vi "NewBusNumber.vi"(8 "ErrorArray In":errorcluster[](array[cluster]), 10 "clFrontPanelControlRefs In":T1) -> (0 "ErrorArray Out":errorcluster[](array[cluster]), 1 "BusNumber":u8, 2 "clFrontPanelControlRefs Out":T1)   [LabVIEW 2014, in "TestFramework.lvlib"]
uses:
  TestFramework.lvlib
  TypeDefs/clFrontPanelControlRefs.ctl
  FGenPlugins/MyPluginBaseClass/TypeDef/PluginParams.ctl
  WfrmGenerator/WfrmPlugins/EventPluginBaseClass/TypeDefs/dblEvtSignalArray.ctl
  FGenPlugins/MyPluginBaseClass/TypeDef/CreateArbWfrmParams.ctl
  WfrmGenerator/WfrmPlugins/EventPluginBaseClass/TypeDefs/clEvtConfig.ctl
  WfrmGenerator/WfrmModule/PublicAPI/Arguments/Requests/dblEvtParams.ctl
  FGenPlugins/MyPluginBaseClass/TypeDef/ConfigArbWfrmParams.ctl
  FGenPlugins/MyPluginBaseClass/TypeDef/TriggerParams.ctl
  <vilib>/Utility/error.llb/Error Cluster From Error Code.vi
  <vilib>/ErrorRing/Error Ring.xnode
  <userlib>/NIST/NISTErrorLib/NISTErrorLib.lvlib
  FGenPlugins/MyPluginBaseClass/NISTFGenPluginsBase.lvclass
  WfrmGenerator/WfrmPlugins/EventPluginBaseClass/BaseWfrmPlugin.lvclass
  WfrmGenerator/WfrmModule/WfrmModule.lvlib
panel:
  # "When you add a control \non the front panel, add a\nreference for it in this\ntype def.  This cluster\nwill hold all of the refer-\nences to the front panel\ncontrols in order to pass\nthese control references \nto subvis."
  # "When you add a control \non the front panel, add a\nreference for it in this\ntype def.  This cluster\nwill hold all of the refer-\nences to the front panel\ncontrols in order to pass\nthese control references \nto subvis."
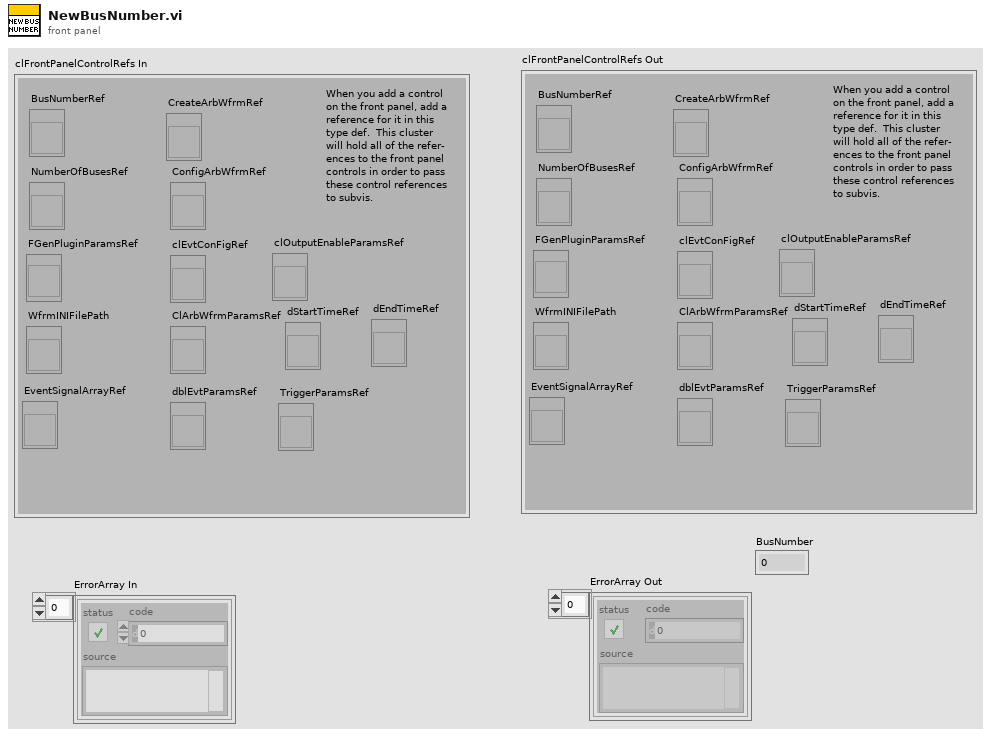
[diagram p1: front panel]
types:
  T1 = typedef "TestFramework.lvlib/clFrontPanelControlRefs.ctl" = cluster{"BusNumberRef":refnum<vi>, "NumberOfBusesRef":refnum<vi>, "FGenPluginParamsRef":refnum<vi>, "WfrmINIFilePath":refnum<vi>, "EventSignalArrayRef":refnum<vi>, "CreateArbWfrmRef":refnum<vi>, "clEvtConFigRef":refnum<vi>, "dblEvtParamsRef":refnum<vi>, "clOutputEnableParamsRef":refnum<vi>, "ConfigArbWfrmRef":refnum<vi>, "ClArbWfrmParamsRef":refnum<vi>, "dStartTimeRef":refnum<vi>, "dEndTimeRef":refnum<vi>, "TriggerParamsRef":refnum<vi>}
  T2 = typedef "LVStringsAndValuesArrayTypeDef_U8.ctl" = cluster{"String":string, "Value":u8}[]
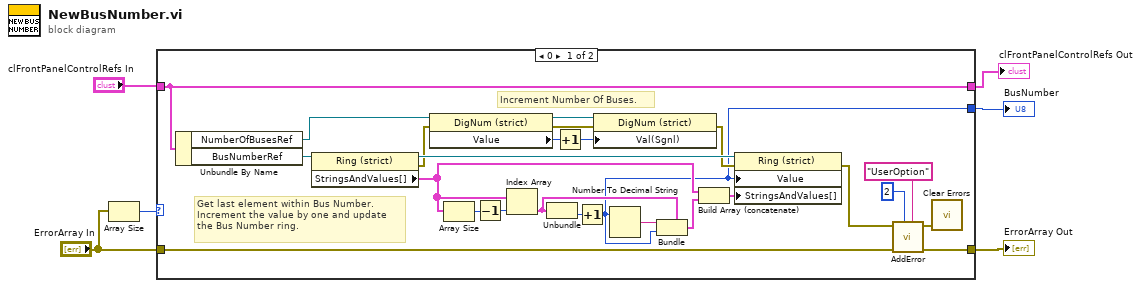
[diagram p0: block diagram]
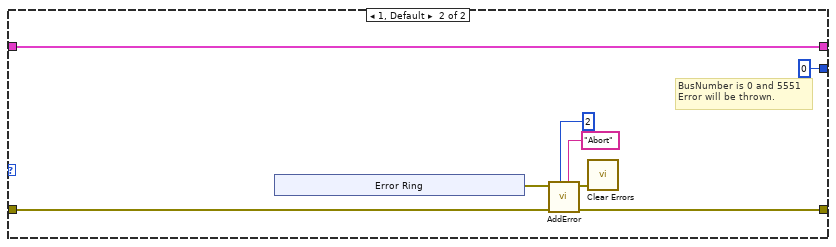
[diagram p2: hidden frame]
diagram:
  n1 = Array Size(array="ErrorArray In") -> (size(s)=w3:i32)
  n2 = case shown="0" w3 {
    tunnel: "clFrontPanelControlRefs In" -> [w23 w39]
    tunnel: [w23 w39] -> w4
    tunnel: [w13 u8 0] -> w5
    tunnel: "ErrorArray In" -> [w8 w33]
    tunnel: [w7 w32] -> w1
    frame 0 {
      # "Get last element within Bus Number.\nIncrement the value by one and update\nthe Bus Number ring."
      # "Increment Number Of Buses."
      n3 = Unbundle By Name(w23) -> ("NumberOfBusesRef"=w27:refnum<vi>, "BusNumberRef"=w26:refnum<vi>)
      n4 = property class="Ring (strict)"(reference=w26) -> (reference out=w28:refnum<vi>, error out=w25:errorcluster, "StringsAndValues[]"=w16:T2)  [unwired: 1 in]
      n5 = property class="DigNum (strict)"(reference=w27, error in=w25) -> (reference out=w30:refnum<vi>, error out=w29:errorcluster, "Value"=w31:u8)
      n6 = Array Size(array=w16) -> (size(s)=w21:i32)
      n7 = Decrement(x=w21) -> (x-1=w20:i32)
      n8 = Index Array(array=w16, index=w20) -> (element=w18:cluster{"String":string, "Value":u8})
      n9 = Unbundle(w18) -> ("Value"=w19:u8)  [unwired: 1 out]
      n10 = Increment(x=w31) -> (x+1=w22:u8)
      n11 = Increment(x=w19) -> (x+1=w13:u8)
      n12 = property class="DigNum (strict)"(reference=w30, error in=w29, "Val(Sgnl)"=w22) -> (error out=w24:errorcluster)  [unwired: 1 out]
      n13 = Number To Decimal String(number=w13) -> (decimal integer string=w17:string)  [unwired: 1 in]
      n14 = Bundle(cluster=w18, "String"=w17, "Value"=w13) -> (w15:cluster{"String":string, "Value":u8})
      n15 = Build Array (concatenate)(w16, w15) -> (w14:T2)
      n16 = property class="Ring (strict)"(reference=w28, error in=w24, "Value"=w13, "StringsAndValues[]"=w14) -> (error out=w9:errorcluster)  [unwired: 1 out]
      n17 = call <userlib>:"AddError.vi"("Severity"="UserOption" ("String"), "Priority"=u8 2, "ErrorArray"=w8, "error in (no error)"=w9) -> ("ErrorArray"=w7:errorcluster[], "error out"=w12:errorcluster)  [unwired: 6 in]
      n18 = call <vilib>:"Clear Errors.vi"("error in (no error)"=w12) -> ()  [unwired: 5 in, 2 out]
    }
    frame 1, Default {
      # "BusNumber is 0 and 5551\nError will be thrown."
      n19 = xnode "Error Ring"() -> ("error out"=w34:errorcluster)
      n20 = call <userlib>:"AddError.vi"("Severity"="Abort" ("String"), "Priority"=u8 2, "ErrorArray"=w33, "error in (no error)"=w34) -> ("ErrorArray"=w32:errorcluster[], "error out"=w37:errorcluster)  [unwired: 6 in]
      n21 = call <vilib>:"Clear Errors.vi"("error in (no error)"=w37) -> ()  [unwired: 5 in, 2 out]
    }
  }
  "BusNumber" <- w5
  "clFrontPanelControlRefs Out" <- w4
  "ErrorArray Out" <- w1
